vi "Check_motor_comm.VI"(1 "Number of Lines before":i32, 5 "Serial read string concat":string) -> (2 "Number of Lines found current":i32, 3 "Read  strings arr":string[](array[string]), 4 "Number of Steps Made":i32, 6 "Command received?":bool, 8 "Move complete?":bool, 10 "com_fail":bool)   [LabVIEW 2019]
panel:
  out "after substring":string
  out "String Array Matched":string[](array[string])=["c:\\DATA\\20141011-102717-0.fits", "c:\\DATA\\20141011-102717-1.fits"]
  out "Values 2":string[](array[string])
  out "Values found":string[][](array[string])
  out "Vallue found?":bool[](array[boolean])
  out "Values  arr size(s)":i32
  out "Str found?":bool[](array[boolean])
  out "Values":string[](array[string])
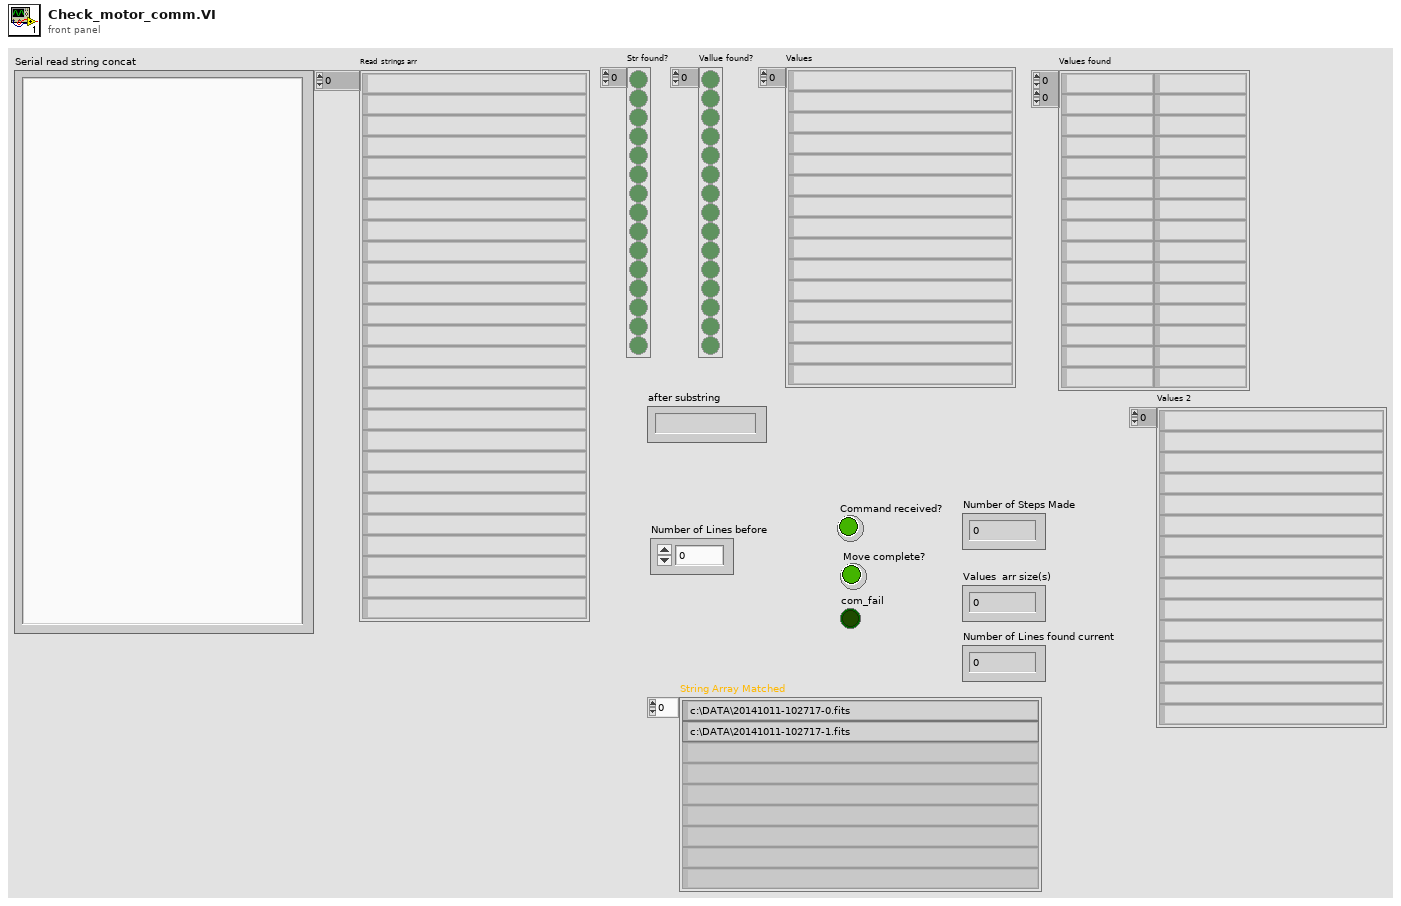
[diagram p1: front panel]
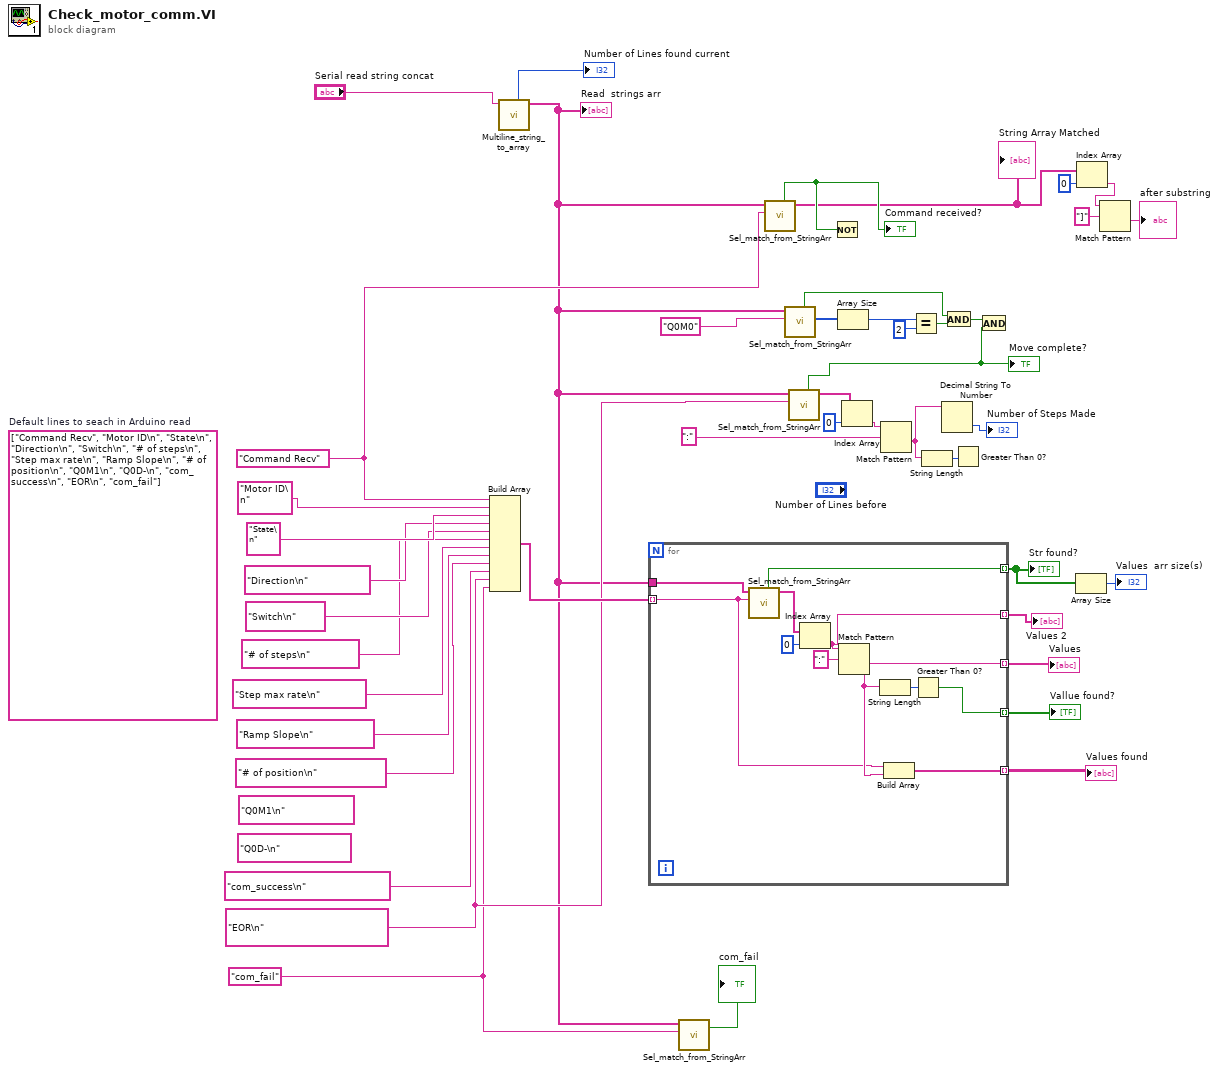
[diagram p0: block diagram]
diagram:
  w2 = "com_fail"
  w21 = "EOR\n"
  (unwired) "Q0D-\n"
  (unwired) "Q0M1\n"
  w16 = "Command Recv"
  (unwired) string[] ["Command Recv", "Motor ID\n", "State\n", "Direction\n", "Switch\n", "# of steps\n", "Step max rate\n", "Ramp Slope\n", "# of position\n", "Q0M1\n", "Q0D-\n", "com_success\n", "EOR\n", "com_fail"]  # Default lines to seach in Arduino read
  n1 = Build Array(w16, "Motor ID\n", "State\n", "Direction\n", "Switch\n", "# of steps\n", "Step max rate\n", "Ramp Slope\n", "# of position\n", "com_success\n", w21, w2) -> (w22:string[])
  n2 = call "Multiline_string_to_array.vi"("Input string"="Serial read string concat") -> ("String Array Out"=w3:string[], "Number of LF matches"=→"Number of Lines found current":i32)  [unwired: 7 in, 2 out]
  "Read  strings arr" <- w3
  n3 = for {
    tunnel: w3 -> [w55]
    tunnel: w22 -> [w47] mode=indexing
    tunnel: [w54] -> w34 mode=indexing
    tunnel: [w48] -> w35 mode=indexing
    tunnel: [w49] -> w23 mode=indexing
    tunnel: [w46] -> w10 mode=indexing
    tunnel: [w45] -> w9 mode=indexing
    n4 = call "Sel_match_from_StringArr.vi"("String to match"=w47, "String Array In"=w55) -> ("String Array Matched"=w53:string[], "Str found?"=w54:bool)  [unwired: 6 in, 2 out]
    n5 = Index Array(array=w53, index=0) -> (element=w45:string)
    n6 = Match Pattern(string=w45, regular expression=":") -> (after substring=w48:string)  [unwired: 1 in, 3 out]
    n7 = String Length(string=w48) -> (length=w50:i32)
    n8 = Build Array(w47, w48) -> (w46:string[])
    n9 = Greater Than 0?(x=w50) -> (x > 0?=w49:bool)
  }
  "Values" <- w35
  "Str found?" <- w34
  "Vallue found?" <- w23
  "Values found" <- w10
  "Values 2" <- w9
  n10 = call "Sel_match_from_StringArr.vi"("String to match"=w2, "String Array In"=w3) -> ("Str found?"=→"com_fail":bool)  [unwired: 6 in, 3 out]
  n11 = call "Sel_match_from_StringArr.vi"("String to match"=w16, "String Array In"=w3) -> ("String Array Matched"=w5:string[], "Str found?"=w12:bool)  [unwired: 6 in, 2 out]
  "Command received?" <- w12
  "String Array Matched" <- w5
  n12 = call "Sel_match_from_StringArr.vi"("String to match"="Q0M0", "String Array In"=w3) -> ("Inx matches"=w40:i32[], "Str found?"=w39:bool)  [unwired: 6 in, 2 out]
  n13 = call "Sel_match_from_StringArr.vi"("String to match"=w21, "String Array In"=w3) -> ("String Array Matched"=w17:string[], "Str found?"=w11:bool)  [unwired: 6 in, 2 out]
  "Move complete?" <- w11
  n14 = Not(x=w12) -> ()  [unwired: 1 out]
  n15 = Array Size(array=w40) -> (size(s)=w41:i32)
  n16 = Index Array(array=w17, index=0) -> (element=w19:string)
  n17 = Match Pattern(string=w19, regular expression=":") -> (after substring=w14:string)  [unwired: 1 in, 3 out]
  n18 = Equal?(x=w41, y=2) -> (x = y?=w44:bool)
  n19 = String Length(string=w14) -> (length=w15:i32)
  n20 = Decimal String To Number(string=w14) -> (number=→"Number of Steps Made":i32)  [unwired: 2 in, 1 out]
  n21 = And(x=w39, y=w44) -> (x .and. y?=w43:bool)
  n22 = Greater Than 0?(x=w15) -> ()  [unwired: 1 out]
  n23 = And(x=w43, y=w11) -> ()  [unwired: 1 out]
  n24 = Array Size(array=w34) -> (size(s)=→"Values  arr size(s)":i32)
  n25 = Index Array(array=w5, index=0) -> (element=w6:string)
  n26 = Match Pattern(string=w6, regular expression="]") -> (after substring=→"after substring":string)  [unwired: 1 in, 3 out]
